vi "XY graph cursor_0127.vi"() -> ()   [LabVIEW 2021]
uses:
  <vilib>/Utility/miscctls.llb/LVCursorListTypeDef.ctl
panel:
  out "Waveform Graph":dbl[][](graph)
  in  "Plot1 Y-Offset":dbl
  in  "Plot1  X-Offset":dbl
  in  "Plot1 Style":u8=4
  in  "Plot1 Point Style":u8=13
  in  "Plot 0  Y-Offset":dbl
  in  "Plot 0 X-Offset":dbl
  in  "Plot 0 Style":u8
  in  "Plot 0 Point Style":u8
  in  "Cursor List":T1=[{"Name"="", "Color"=0, "Style"=0, "Point Style"=0, "Name Visible"=TRUE, "Allow Drag"=FALSE, "Cursor Mode"=0, "Plot"=0, "Index"=0, "Position"={"X"=0.0, "Y"=0.0}, "X Scale"=0, "Y Scale"=0, "Watch Plots"=[], "Watch All Plots"=FALSE, "Plot Area"=0, "Label Offset"={"X"=8.0, "Y"=0.05}}]
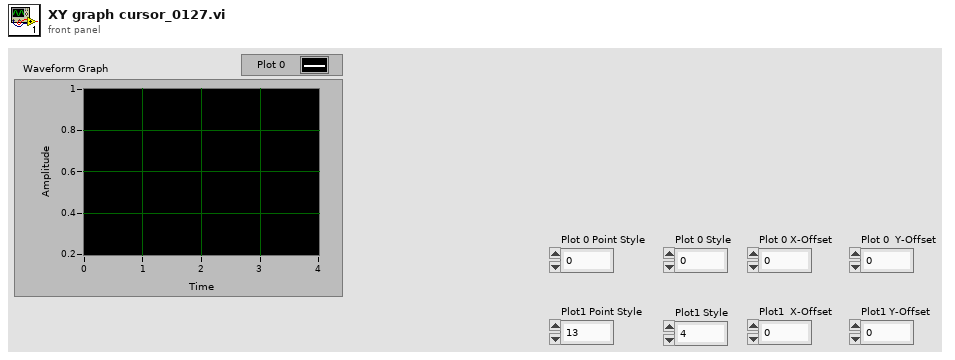
[diagram p1: front panel]
types:
  T1 = typedef "LVCursorListTypeDef.ctl" = cluster{"Name":string, "Color":u32, "Style":u8, "Point Style":u8, "Name Visible":bool, "Allow Drag":bool, "Cursor Mode":u32, "Plot":i32, "Index":i32, "Position":cluster{"X":dbl, "Y":dbl}, "X Scale":u32, "Y Scale":u32, "Watch Plots":i32[], "Watch All Plots":bool, "Plot Area":i32, "Label Offset":cluster{"X":dbl, "Y":dbl}}[]
  T2 = cluster{"Name":string, "Color":u32, "Style":u8, "Point Style":u8, "Name Visible":bool, "Allow Drag":bool, "Cursor Mode":u32, "Plot":i32, "Index":i32, "Position":cluster{"X":dbl, "Y":dbl}, "X Scale":u32, "Y Scale":u32, "Watch Plots":i32[], "Watch All Plots":bool, "Plot Area":i32, "Label Offset":cluster{"X":dbl, "Y":dbl}}
  T3 = cluster{"Name":string, "Color":u32, "Style":u8, "Point Style":u8, "Name Visible":bool, "Allow Drag":bool, "Cursor Mode":u32, "Plot":i32, "Index":i32, "Position":cluster{"X":dbl, "Y":dbl}, "X Scale":u32, "Y Scale":u32, "Watch Plots":i32[], "Watch All Plots":bool, "Plot Area":i32, "Label Offset":cluster{"X":dbl, "Y":dbl}}[]
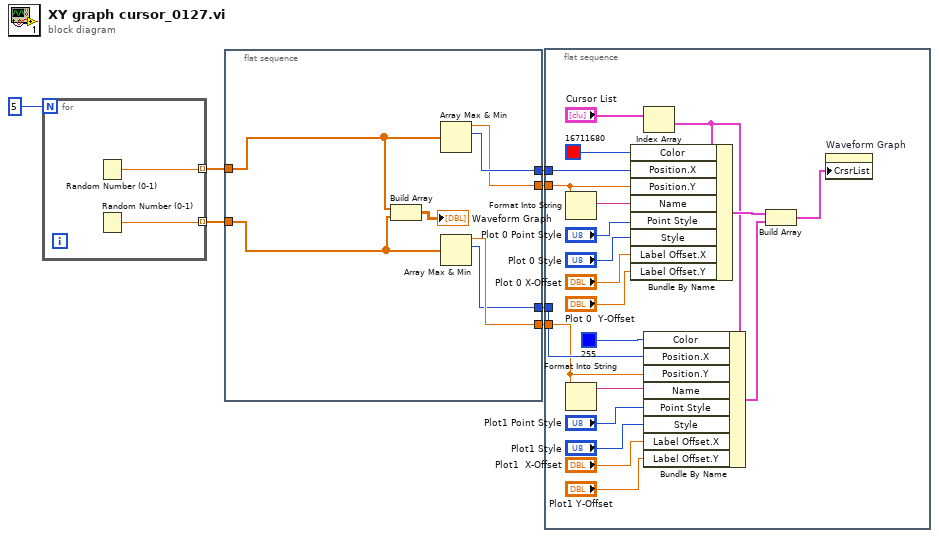
[diagram p0: block diagram]
diagram:
  n1 = for {
    N: 5 -> [_]
    tunnel: [w9] -> w4 mode=indexing
    tunnel: [w8] -> w3 mode=indexing
    n2 = Random Number (0-1)() -> (number: 0 to 1=w9:dbl)
    n3 = Random Number (0-1)() -> (number: 0 to 1=w8:dbl)
  }
  n4 = flat-sequence {
    tunnel: [w16] -> w6
    tunnel: [w15] -> w5
    tunnel: w4 -> [w12]
    tunnel: w3 -> [w11]
    tunnel: [w14] -> w2
    tunnel: [w13] -> w1
    frame #0 {
      n5 = Build Array(w12, w11) -> (→"Waveform Graph":dbl[][])
      n6 = Array Max & Min(array=w12) -> (max value=w15:dbl, max index (indices)=w16:i32)  [unwired: 2 out]
      n7 = Array Max & Min(array=w11) -> (max value=w14:dbl, max index (indices)=w13:i32)  [unwired: 2 out]
    }
  }
  n8 = flat-sequence {
    tunnel: w6 -> [w34]
    tunnel: w5 -> [w32]
    tunnel: w2 -> [w26]
    tunnel: w1 -> [w27]
    frame #0 {
      n9 = Format Into String(w32) -> (resulting string=w33:string)  [unwired: 3 in, 1 out]
      n10 = Format Into String(w26) -> (resulting string=w29:string)  [unwired: 3 in, 1 out]
      n11 = Index Array(array="Cursor List") -> (element=w25:T2)  [unwired: 1 in]
      n12 = Bundle By Name(cluster=w25, "Color"=u32 16711680, "Position.X"=w34, "Position.Y"=w32, "Name"=w33, "Point Style"="Plot 0 Point Style", "Style"="Plot 0 Style", "Label Offset.X"="Plot 0 X-Offset", "Label Offset.Y"="Plot 0  Y-Offset") -> (w36:T2)
      n13 = Bundle By Name(cluster=w25, "Color"=u32 255, "Position.X"=w27, "Position.Y"=w26, "Name"=w29, "Point Style"="Plot1 Point Style", "Style"="Plot1 Style", "Label Offset.X"="Plot1  X-Offset", "Label Offset.Y"="Plot1 Y-Offset") -> (w24:T2)
      n14 = Build Array(w36, w24) -> (w17:T3)
      n15 = property on="Waveform Graph" class="WFGraph (strict)"("CrsrList"=w17) -> ()  [unwired: 2 in, 2 out]
    }
  }
